vi "TcpCommunicationClientModule.vi"(7 "TcpCommunicationClientCMD":T1, 8 "エラー入力（エラーなし）":errorcluster, 9 "WriteData":string, 10 "ポート":u16, 11 "アドレス":string) -> (0 "エラー出力":errorcluster, 1 "Data":string, 2 "Command":string, 4 "TcpOK?":bool, 5 "ReadData":string)   [LabVIEW 2021]
doc: "クライアント用TCP通信モジュール\nRead　：データの受信を行い、ReadDataに出力します。スペースを区切りにCommandとDataを分けます。\nWrite　：データの送信を行います。WriteDataの文字列の末尾にCRを加えて送信します。\nClose　：通信を閉じます。"
uses:
  TcpCommunicationClientCMD.ctl
panel:
  # "クライアント用TCP通信モジュール"
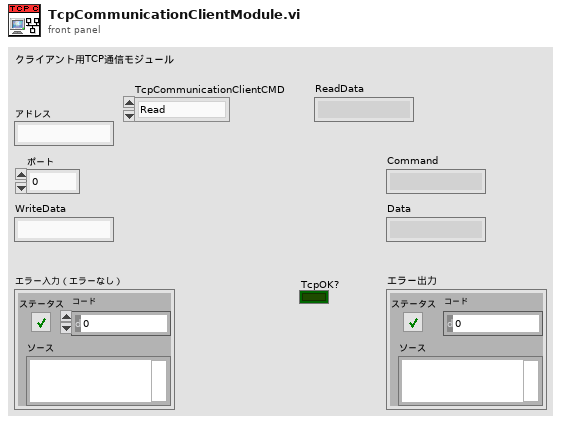
[diagram p1: front panel]
types:
  T1 = typedef "TcpCommunicationClientCMD.ctl" = enum16{"Read", "Write", "Close"}
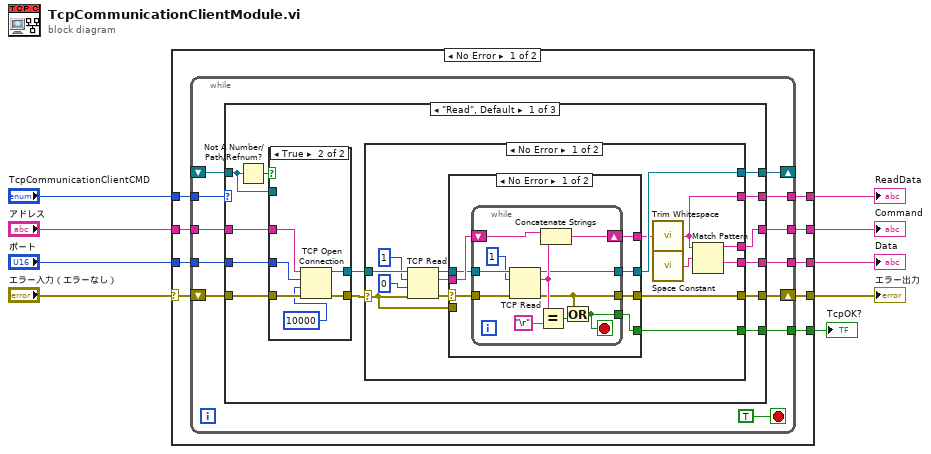
[diagram p0: block diagram]
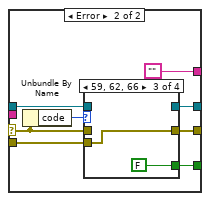
[diagram p2: hidden frame]
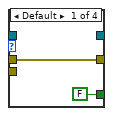
[diagram p3: hidden frame]
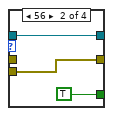
[diagram p4: hidden frame]
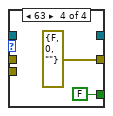
[diagram p5: hidden frame]
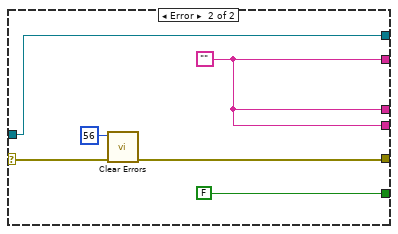
[diagram p6: hidden frame]
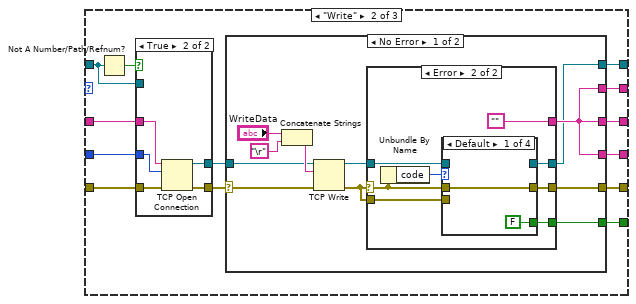
[diagram p8: hidden frame]
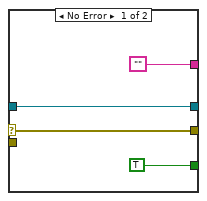
[diagram p9: hidden frame]
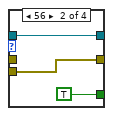
[diagram p10: hidden frame]
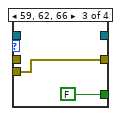
[diagram p11: hidden frame]
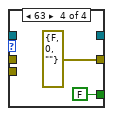
[diagram p12: hidden frame]
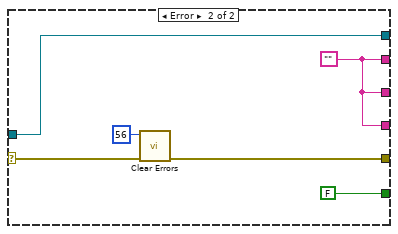
[diagram p13: hidden frame]
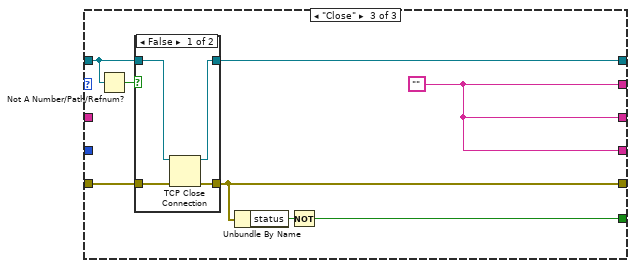
[diagram p15: hidden frame]
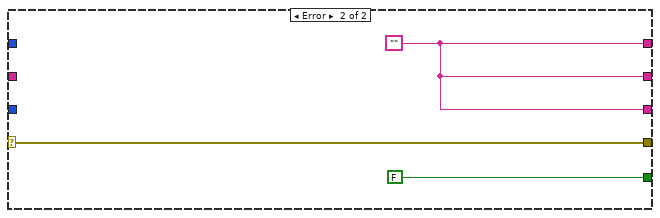
[diagram p17: hidden frame]
diagram:
  n1 = case shown="No Error" "エラー入力（エラーなし）" {
    selector: "エラー入力（エラーなし）" -> [w14 w182]
    tunnel: "ポート" -> [w18 _]
    tunnel: "アドレス" -> [w17 _]
    tunnel: [w16 w182] -> w7
    tunnel: [w15 w181] -> w6
    tunnel: "TcpCommunicationClientCMD" -> [w13 _]
    tunnel: [w12 w181] -> w3
    tunnel: [w11 w181] -> w2
    tunnel: [w10 FALSE] -> w1
    frame No Error {
      n2 = while {
        tunnel: w18 -> [w30]
        tunnel: w17 -> [w29]
        tunnel: [w27] -> w15
        shift-right: [w28] -> w16
        shift-left: w14 -> [w26]
        shift-right: [w24] -> _
        shift-left: _ -> [w23]
        tunnel: w13 -> [w22]
        tunnel: [w21] -> w12
        tunnel: [w20] -> w11
        tunnel: [w19] -> w10
        stop <- TRUE stop-if-true
        n3 = case shown="\"Read\", Default" w22 {
          tunnel: w30 -> [w43 w117 _]
          tunnel: w29 -> [w42 w118 _]
          tunnel: [w39 w112 w168] -> w28
          tunnel: [w33 w113 w169] -> w27
          tunnel: w26 -> [w38 w116 w172]
          tunnel: [w37 w114 w170] -> w24
          tunnel: w23 -> [w36 w119 w171]
          tunnel: [w35 w109 w169] -> w21
          tunnel: [w34 w108 w169] -> w20
          tunnel: [w32 w111 w166] -> w19
          frame "Read", Default {
            n4 = Not A Number/Path/Refnum?(number/path/refnum=w36) -> (NaN/Path/Refnum?=w41:bool)
            n5 = case shown="True" w41 {
              tunnel: [w100 w107] -> w40
              tunnel: [w101 w103] -> w31
              tunnel: w38 -> [w101 w106]
              tunnel: w36 -> [w100 _]
              tunnel: w42 -> [_ w105]
              tunnel: w43 -> [_ w104]
              frame False {
              }
              frame True {
                n6 = TCP Open Connection(address=w105, remote port or service name=w104, timeout ms (60000)=10000, error in (no error)=w106) -> (connection ID=w107:refnum<k5>, error out=w103:errorcluster)  [unwired: 1 out]
              }
            }
            n7 = case shown="No Error" w31 {
              selector: w31 -> [w44 w97]
              tunnel: w40 -> [w58 w99]
              tunnel: [w57 w95] -> w39
              tunnel: [w56 w99] -> w37
              tunnel: [w48 w98] -> w35
              tunnel: [w47 w98] -> w34
              tunnel: [w46 w98] -> w33
              tunnel: [w45 FALSE] -> w32
              frame No Error {
                n8 = TCP Read(connection ID=w58, bytes to read=1 ("読み取りバイト数"), error in (no error)=w44, 9:0 ("タイムアウト")) -> (connection ID out=w53:refnum<k5>, data out=w51:string, error out=w52:errorcluster)  [unwired: 1 out]
                n9 = case shown="No Error" w52 {
                  selector: w52 -> [w63 w83]
                  tunnel: w53 -> [w64 w81]
                  tunnel: w51 -> [w65 _]
                  tunnel: w44 -> [_ w82]
                  tunnel: [w62 w80] -> w57
                  tunnel: [w61 w79] -> w56
                  tunnel: [w60 ""] -> w49
                  tunnel: [w59 w77] -> w45
                  frame No Error {
                    # "クライアントがデータを送信した場合、接続を閉じる必要があることを示しています。"
                    n10 = while {
                      shift-right: [w68] -> w60
                      shift-left: w65 -> [w72]
                      tunnel: w64 -> [w76]
                      tunnel: w63 -> [w75]
                      tunnel: [w67] -> w62
                      tunnel: [w70] -> w61
                      tunnel: [w66] -> w59
                      stop <- w66 stop-if-true
                      n11 = TCP Read(connection ID=w76, bytes to read=1 ("読み取りバイト数"), error in (no error)=w75) -> (connection ID out=w70:refnum<k5>, data out=w71:string, error out=w67:errorcluster)  [unwired: 1 in, 1 out]
                      n12 = Equal?(x=w71, y="\r") -> (x = y?=w69:bool)
                      n13 = Concatenate Strings(w72, w71) -> (w68:string)
                      n14 = Or(x=w67, y=w69) -> (x .or. y?=w66:bool)
                    }
                  }
                  frame Error {
                    # "閉じられた接続とタイムアウトエラーを無視する"
                    n15 = Unbundle By Name(w83) -> ("code"=w84:i32)
                    n16 = case shown="59, 62, 66" w84 {
                      tunnel: w83 -> [w86 _ _ _]
                      tunnel: [w86 w88 w91 errorcluster {"status"=FALSE, "code"=0, "source"=""} ("error out")] -> w80
                      tunnel: w82 -> [_ w88 w91 _]
                      tunnel: w81 -> [_ w89 _ _]
                      tunnel: [_ w89 _ _] -> w79
                      tunnel: [FALSE TRUE FALSE FALSE] -> w77
                      frame Default {
                        # "不明なエラーのため渡してください。"
                      }
                      frame 56 {
                        # "「TCP読み取り」関数がタイムアウトした場合、接続は依然有効であるため現在のデータをクライアントに送信することができます。データに文字列長を追加して、クライアントに読み取りバイト数を知らせます。"
                      }
                      frame 59, 62, 66 {
                        # "接続が閉じたため、このクライアントrefnumは無効になりました。"
                      }
                      frame 63 {
                      }
                    }
                  }
                }
                n17 = call <vilib>:"Trim Whitespace.vi"("string"=w49) -> ("trimmed string"=w46:string)  [unwired: 1 in]
                n18 = call <vilib>:"Space Constant.vi"() -> ("String"=w50:string)
                n19 = Match Pattern(string=w46, regular expression=w50) -> (before substring=w48:string, after substring=w47:string)  [unwired: 1 in, 2 out]
              }
              frame Error {
                w98 = ""
                n20 = call <vilib>:"Clear Errors.vi"("error in (no error)"=w97, "specific error code to clear (0: all)"=56) -> ("error out"=w95:errorcluster)  [unwired: 4 in, 1 out]
              }
            }
          }
          frame "Write" {
            n21 = Not A Number/Path/Refnum?(number/path/refnum=w119) -> (NaN/Path/Refnum?=w120:bool)
            n22 = case shown="True" w120 {
              tunnel: [w159 w165] -> w115
              tunnel: [w160 w164] -> w110
              tunnel: w116 -> [w160 w163]
              tunnel: w119 -> [w159 _]
              tunnel: w118 -> [_ w162]
              tunnel: w117 -> [_ w161]
              frame False {
              }
              frame True {
                n23 = TCP Open Connection(address=w162, remote port or service name=w161, error in (no error)=w163) -> (connection ID=w165:refnum<k5>, error out=w164:errorcluster)  [unwired: 2 out]
              }
            }
            n24 = case shown="No Error" w110 {
              selector: w110 -> [w127 w158]
              tunnel: w115 -> [w129 w154]
              tunnel: [w124 w154] -> w114
              tunnel: [w125 w153] -> w113
              tunnel: [w121 w157] -> w112
              tunnel: [w126 FALSE] -> w111
              tunnel: [w125 w153] -> w109
              tunnel: [w125 w153] -> w108
              frame No Error {
                n25 = Concatenate Strings("WriteData", "\r") -> (w131:string)
                n26 = TCP Write(connection ID=w129, data in=w131, error in (no error)=w127) -> (connection ID out=w122:refnum<k5>, error out=w123:errorcluster)  [unwired: 1 in, 1 out]
                n27 = case shown="Error" w123 {
                  selector: w123 -> [w135 w142]
                  tunnel: w122 -> [w133 w140]
                  tunnel: w123 -> [_ w141]
                  tunnel: [w135 w139] -> w121
                  tunnel: [w133 w138] -> w124
                  tunnel: ["" ""] -> w125
                  tunnel: [TRUE w136] -> w126
                  frame No Error {
                    # "クライアントがデータを送信した場合、接続を閉じる必要があることを示しています。"
                  }
                  frame Error {
                    # "閉じられた接続とタイムアウトエラーを無視する"
                    n28 = Unbundle By Name(w142) -> ("code"=w143:i32)
                    n29 = case shown="Default" w143 {
                      tunnel: w142 -> [w145 _ _ _]
                      tunnel: [w145 w147 w150 errorcluster {"status"=FALSE, "code"=0, "source"=""} ("error out")] -> w139
                      tunnel: w141 -> [_ w147 w150 _]
                      tunnel: w140 -> [_ w148 _ _]
                      tunnel: [_ w148 _ _] -> w138
                      tunnel: [FALSE TRUE FALSE FALSE] -> w136
                      frame Default {
                        # "不明なエラーのため渡してください。"
                      }
                      frame 56 {
                        # "「TCP読み取り」関数がタイムアウトした場合、接続は依然有効であるため現在のデータをクライアントに送信することができます。データに文字列長を追加して、クライアントに読み取りバイト数を知らせます。"
                      }
                      frame 59, 62, 66 {
                        # "接続が閉じたため、このクライアントrefnumは無効になりました。"
                      }
                      frame 63 {
                      }
                    }
                  }
                }
              }
              frame Error {
                w153 = ""
                n30 = call <vilib>:"Clear Errors.vi"("error in (no error)"=w158, "specific error code to clear (0: all)"=56) -> ("error out"=w157:errorcluster)  [unwired: 4 in, 1 out]
              }
            }
          }
          frame "Close" {
            w169 = ""
            n31 = Not A Number/Path/Refnum?(number/path/refnum=w171) -> (NaN/Path/Refnum?=w173:bool)
            n32 = case shown="False" w173 {
              tunnel: [w174 w178] -> w170
              tunnel: [w176 w179] -> w168
              tunnel: w172 -> [w177 w179]
              tunnel: w171 -> [w175 w178]
              frame False {
                n33 = TCP Close Connection(connection ID=w175, error in (no error)=w177) -> (connection ID out=w174:refnum<k5>, error out=w176:errorcluster)  [unwired: 1 out]
              }
              frame True {
              }
            }
            n34 = Unbundle By Name(w168) -> ("status"=w167:bool)
            n35 = Not(x=w167) -> (.not. x?=w166:bool)
          }
        }
      }
    }
    frame Error {
      w181 = ""
    }
  }
  "エラー出力" <- w7
  "ReadData" <- w6
  "Command" <- w3
  "Data" <- w2
  "TcpOK?" <- w1
